vi "OpenSession.vi"(8 "error in (no error)":errorcluster, 10 "gRPCid":T2, 11 "ctet_dmm":T1) -> (0 "error out":errorcluster, 3 "ctet_dmm out":T1)   [LabVIEW 2019, in "ctet_dmm User Library.lvlib"]
uses:
  Servers/ctet_dmm/gRPC lvSupport/Server API/typeDefs/grpcId.ctl
  Types/ctet_dmm.ctl
  Servers/ctet_dmm/ctet_dmm Class/RPC Messages/measurementservice_DMMOpenSessionResponse/measurementservice_DMMOpenSessionResponse_Data.ctl
  Servers/ctet_dmm/ctet_dmm Class/RPC Messages/measurementservice_ErrorOut/measurementservice_ErrorOut_Data.ctl
  ctet_dmm User Library.lvlib
  Servers/ctet_dmm/ctet_dmm Class/ctet_dmm.lvclass
  Servers/ctet_dmm/gRPC lvSupport/gprc-lvsupport.lvlib
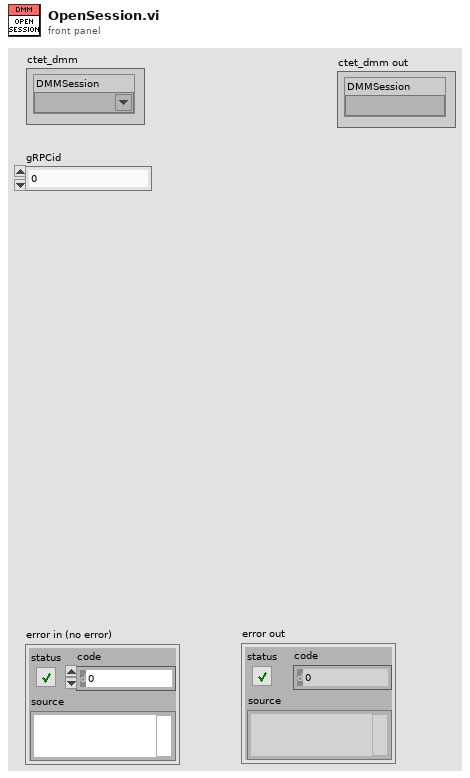
[diagram p1: front panel]
types:
  T1 = typedef "ctet_dmm User Library.lvlib/ctet_dmm.ctl" = cluster{"DMMSession":refnum<k15>}
  T2 = typedef "ctet_dmm.lvlib/gprc-lvsupport.lvlib/grpcId.ctl" = u64
  T3 = typedef "ctet_dmm.lvlib/ctet_dmm.lvclass/measurementservice_ErrorOut_Data.ctl" = cluster{"errCode":i64, "errMessage":string}
  T4 = typedef "ctet_dmm.lvlib/ctet_dmm.lvclass/measurementservice_DMMOpenSessionResponse_Data.ctl" = cluster{"error":T3}
  T5 = typedef "ctet_dmm.lvlib/ctet_dmm.lvclass/measurementservice_DMMOpenSessionRequest_Data.ctl" = cluster{"DMMName":string}
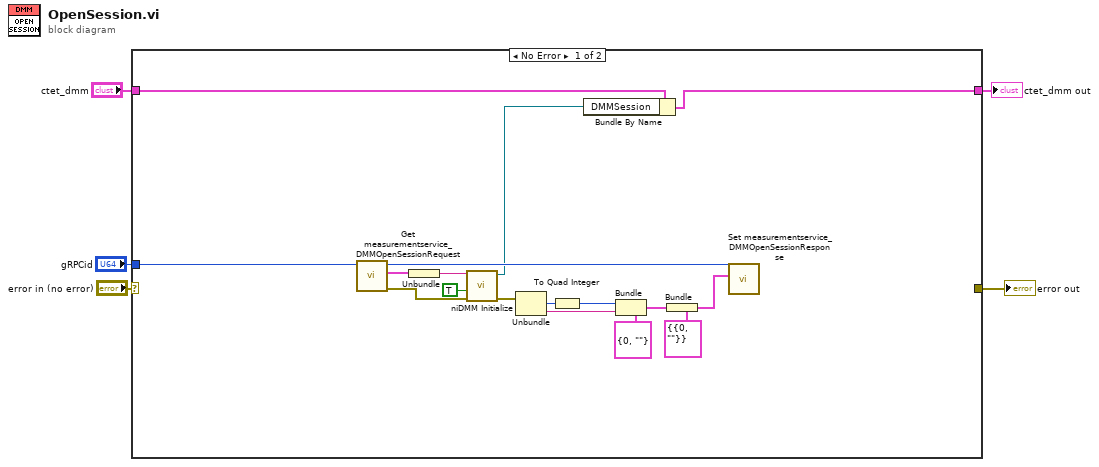
[diagram p0: block diagram]
diagram:
  n1 = case shown="No Error" "error in (no error)" {
    selector: "error in (no error)" -> [_ w24]
    tunnel: [_ w24] -> w5
    tunnel: "gRPCid" -> [w22 _]
    tunnel: "ctet_dmm" -> [w9 w23]
    tunnel: [w7 w23] -> w1
    frame No Error {
      n2 = call "Get measurementservice_DMMOpenSessionRequest.vi"("gRPCid"=w22) -> ("error out"=w6:errorcluster, "Message Data"=w21:T5, "gRPCid out"=w17:T2)  [unwired: 8 in]
      n3 = Unbundle(w21) -> ("DMMName"=w20:string)
      n4 = call <instrlib>:"niDMM Initialize.vi"("error in (no error)"=w6, "Reset"=TRUE, "Instrument Descriptor"=w20) -> ("error out"=w18:errorcluster, "instrument handle out"=w8:refnum<k15>)  [unwired: 7 in]
      n5 = Unbundle(w18) -> ("code"=w11:i32, "source"=w12:string)  [unwired: 1 out]
      n6 = To Quad Integer(1:w11) -> (0:w10:i64)
      n7 = Bundle By Name(cluster=w9, "DMMSession"=w8) -> (w7:T1)
      n8 = Bundle(cluster=T3 {"errCode"=0, "errMessage"=""} ("error"), "errCode"=w10, "errMessage"=w12) -> (w13:T3)
      n9 = Bundle(cluster=T4 {"error"={"errCode"=0, "errMessage"=""}} ("Message Data"), "error"=w13) -> (w15:T4)
      n10 = call "Set measurementservice_DMMOpenSessionResponse.vi"("Message Data"=w15, "gRPCid"=w17) -> ()  [unwired: 9 in, 1 out]
    }
    frame Error {
    }
  }
  "error out" <- w5
  "ctet_dmm out" <- w1
